vi "onSubscribe.vi"(6 "timeout (1000ms)":i32=1000, 8 "error in (no error)":errorcluster, 10 "SUBSCRIBE":refnum<class "SUBSCRIBE.lvclass">, 11 "Client in":refnum<class "Client.lvclass">) -> (0 "error out":errorcluster, 1 "Ack?":bool, 2 "SUBACK":refnum<class "SUBACK.lvclass">, 3 "Client out":refnum<class "Client.lvclass">)   [LabVIEW 2013, in "MQTT Client.lvlib" / "Client.lvclass"]
uses:
  Client.lvclass
  <vilib>/LabVIEW Open Source Project/MQTT Control Packets/Control Packets/SUBSCRIBE/SUBSCRIBE.lvclass
  <vilib>/LabVIEW Open Source Project/MQTT Control Packets/Control Packets/SUBACK/SUBACK.lvclass
  <vilib>/LabVIEW Open Source Project/MQTT Control Packets/Control Packets/ControlPacket/ControlPacket.lvclass/ControlPacket.ctl
  Session.Client/Session.Client.lvclass
  <vilib>/LabVIEW Open Source Project/MQTT Control Packets/Control Packets/ControlPacket/ControlPacket.lvclass
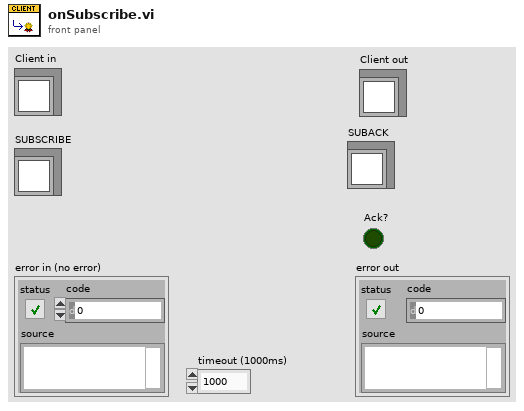
[diagram p1: front panel]
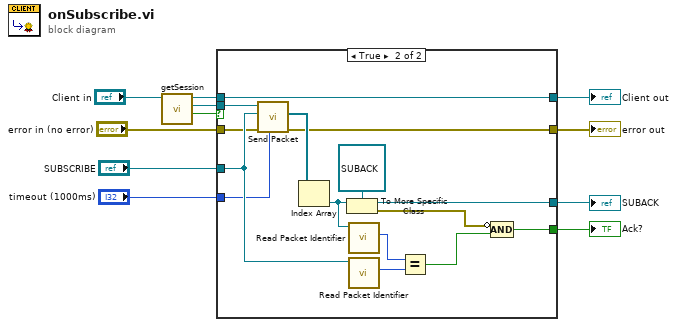
[diagram p0: block diagram]
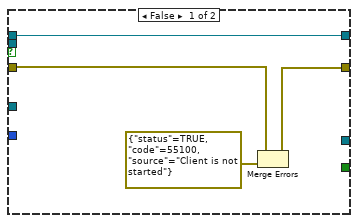
[diagram p2: hidden frame]
diagram:
  n1 = call "getSession.vi"("Client in"="Client in") -> ("valid?"=w2:bool, "Session"=w1:refnum<class "Session.Client.lvclass">, "Client out"=w3:refnum<class "Client.lvclass">)  [unwired: 8 in]
  n2 = case shown="True" w2 {
    tunnel: [w12 w20] -> w11
    tunnel: "error in (no error)" -> [w14 w18]
    tunnel: [w13 w17] -> w9
    tunnel: "timeout (1000ms)" -> [_ w21]
    tunnel: [_ w29] -> w7
    tunnel: "SUBSCRIBE" -> [_ w27]
    tunnel: [_ w22] -> w5
    tunnel: w3 -> [w12 w20]
    tunnel: w1 -> [_ w19]
    frame False {
      n3 = Merge Errors(w14, errorcluster {"status"=TRUE, "code"=55100, "source"="Client is not started"} ("error in")) -> (w13:errorcluster)
    }
    frame True {
      n4 = call "Send Packet.vi"("timeout (0ms : no ack)"=w21, "error in (no error)"=w18, "Packet"=w27, "Session"=w19) -> ("error out"=w17:errorcluster, "Response"=w30:refnum<class "ControlPacket.lvclass">[])  [unwired: 4 in, 2 out]
      n5 = Index Array(array=w30) -> (element=w26:refnum<class "ControlPacket.lvclass">)  [unwired: 1 in]
      n6 = To More Specific Class(target class=refnum<class "SUBACK.lvclass"> refnum ("SUBACK.lvclass"), reference=w26) -> (specific class reference=w29:refnum<class "SUBACK.lvclass">, error out=w23:errorcluster)  [unwired: 1 in]
      n7 = call <vilib>:"Read Packet Identifier.vi"("ControlPacket in"=w26) -> ("Packet Identifier"=w25:u16)  [unwired: 9 in, 1 out]
      n8 = call <vilib>:"Read Packet Identifier.vi"("ControlPacket in"=w27) -> ("Packet Identifier"=w24:u16)  [unwired: 9 in, 1 out]
      n9 = Equal?(x=w25, y=w24) -> (x = y?=w16:bool)
      n10 = Compound Arithmetic op=AND(invert w23, w16) -> (w22:bool)
    }
  }
  "error out" <- w9
  "Client out" <- w11
  "SUBACK" <- w7
  "Ack?" <- w5
